vi "DegF to DegC.vi"(2 "Input Temperature in Celcius":dbl, 3 "Input Temperature in Fahrenheit":dbl) -> (0 "Output Temperature in Fahrenheit":dbl, 1 "Output Temperature in Celcius":dbl)   [LabVIEW 2020]
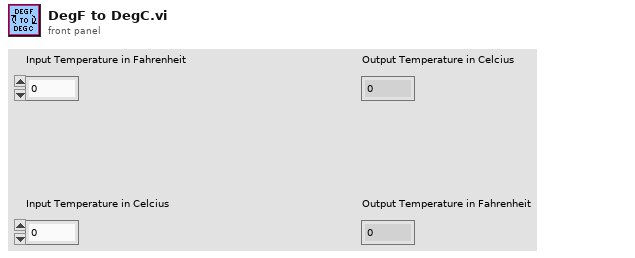
[diagram p1: front panel]
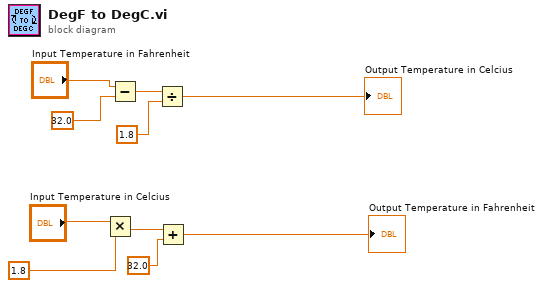
[diagram p0: block diagram]
diagram:
  n1 = Multiply(x="Input Temperature in Celcius", y=1.8) -> (x*y=w3:dbl)
  n2 = Subtract(x="Input Temperature in Fahrenheit", y=32.0) -> (x-y=w8:dbl)
  n3 = Divide(x=w8, y=1.8) -> (x/y=→"Output Temperature in Celcius":dbl)
  n4 = Add(x=w3, y=32.0) -> (x+y=→"Output Temperature in Fahrenheit":dbl)
